vi "Read objChnls.vi"(8 "error in (no error)":errorcluster, 11 "BME_DG_Base in":refnum<class "BME_DG_Base.lvclass">) -> (0 "error out":errorcluster, 1 "DGNr":i32, 2 "objChnls":refnum<class "BME_DG_Chnl.lvclass">[](array[class]), 3 "BME_DG_Base out":refnum<class "BME_DG_Base.lvclass">)   [LabVIEW 2009, in "POLARIS BME DG.lvlib" / "BME_DG_Base.lvclass"]
uses:
  BME_DG_Base.lvclass
  BME_DG_Chnl/BME_DG_Chnl.lvclass
  BME_DG_Base.lvclass/BME_DG_Base.ctl
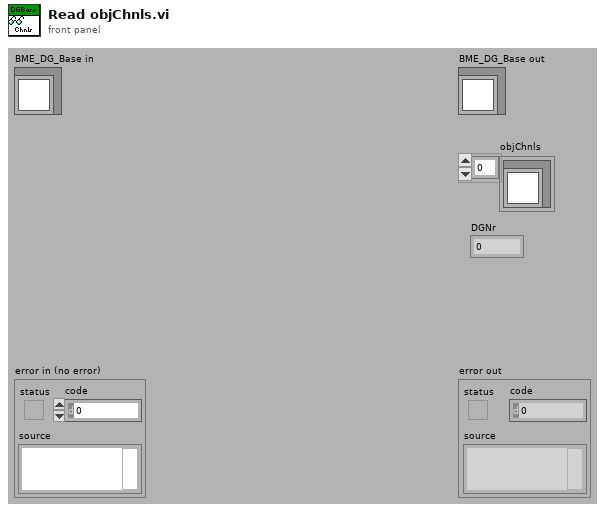
[diagram p1: front panel]
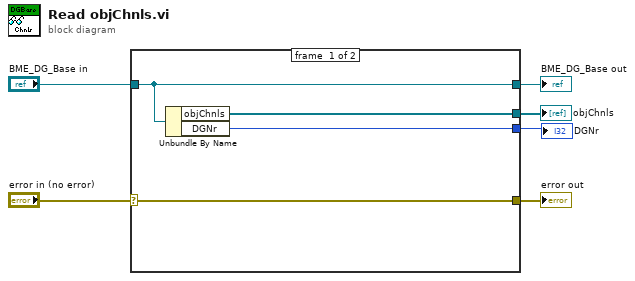
[diagram p0: block diagram]
diagram:
  n1 = case shown="No Error" "error in (no error)" {
    selector: "error in (no error)" -> [w10 w11]
    tunnel: [w10 w11] -> w5
    tunnel: [w9 w12] -> w3
    tunnel: "BME_DG_Base in" -> [w9 w12]
    tunnel: [w8 _] -> w2
    tunnel: [w7 _] -> w1
    frame #0 {
      n2 = Unbundle By Name(w9) -> ("objChnls"=w8:refnum<class "BME_DG_Chnl.lvclass">[], "DGNr"=w7:i32)
    }
    frame #1 {
    }
  }
  "error out" <- w5
  "BME_DG_Base out" <- w3
  "objChnls" <- w2
  "DGNr" <- w1
